vi "Check Keyboard Keys Pressed.vi"(8 "error in (no error)":errorcluster, 10 "key targets (all)":T1(array[ring]), 11 "keys pressed":T1(array[ring])) -> (0 "error out":errorcluster, 2 "keys found":T1(array[ring]), 3 "key found?":bool)   [LabVIEW 2021, in "GUI.lvlib"]
uses:
  GUI.lvlib
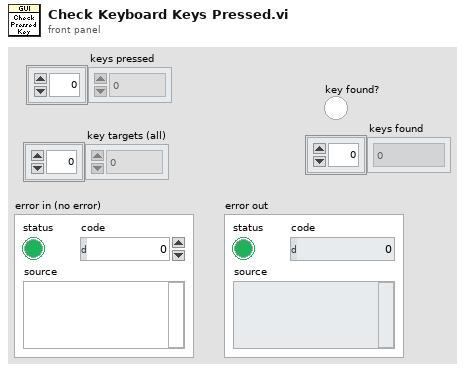
[diagram p1: front panel]
types:
  T1 = enum16{"0", "1", "2", "3", "4", "5", "6", "7", "8", "9", "A", "B", "C", "D", "E", "F", "G", "H", "I", "J", "K", "L", "M", "N", "O", "P", "Q", "R", "S", "T", "U", "V", "W", "X", "Y", "Z", "F1", "F2", "F3", "F4", "F5", "F6", "F7", "F8", "F9", "F10", "F11", "F12", "F13", "F14", "F15", "ADD", "BACK", "BACKSLASH", "CAPITAL", "COMMA", "DECIMAL", "DELETE", "DIVIDE", "DOWN", "END", "EQUALS", "ESCAPE", "GRAVE (`)", "HOME", "INSERT", "LBRACKET", "LCONTROL", "LEFT", "L ALT", "LSHIFT", "LWIN", "MINUS", "MULTIPLY", "NEXT", "NUMLOCK", "NUMPAD_0", "NUMPAD_1", "NUMPAD_2", "NUMPAD_3", "NUMPAD_4", "NUMPAD_5", "NUMPAD_6", "NUMPAD_7", "NUMPAD_8", "NUMPAD_9", "PAUSE", "PERIOD", "PRIOR (PG UP)", "RBRACKET", "RCONTROL", "RETURN", "RIGHT", "R ALT", "RSHIFT", "RWIN", "SCROLL", "SEMICOLON", "SLASH", "SPACE", "SUBTRACT", "TAB", "UP", "ENTER (num pad)", "' (quote)"}[]
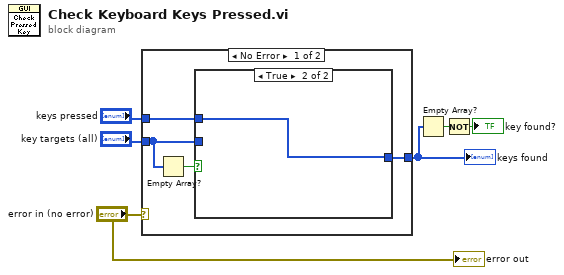
[diagram p0: block diagram]
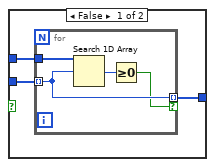
[diagram p2: hidden frame]
diagram:
  n1 = case shown="No Error" "error in (no error)" {
    tunnel: "keys pressed" -> [w10 _]
    tunnel: "key targets (all)" -> [w8 _]
    tunnel: [w9 _] -> w3
    frame No Error {
      n2 = Empty Array?(array=w8) -> (empty?=w7:bool)
      n3 = case shown="True" w7 {
        tunnel: w10 -> [w13 w18]
        tunnel: [w12 w18] -> w9
        tunnel: w8 -> [w11 _]
        frame False {
          n4 = for {
            tunnel: w13 -> [w17]
            tunnel: w11 -> [w16] mode=indexing
            tunnel: [w16] -> w12 mode=indexing if=w14
            n5 = Search 1D Array(1D array=w17, element=w16) -> (index of element=w15:i32)  [unwired: 1 in]
            n6 = Greater Or Equal To 0?(x=w15) -> (x >= 0?=w14:bool)
          }
        }
        frame True {
        }
      }
    }
    frame Error {
    }
  }
  "keys found" <- w3
  n7 = Empty Array?(array=w3) -> (empty?=w2:bool)
  n8 = Not(x=w2) -> (.not. x?=→"key found?":bool)
  "error out" <- "error in (no error)"
